vi "Initialize.vi"(0 "VISA Resource Name":refnum<visa-resource-name>, 5 "ID Query? (T: Yes)":bool=TRUE, 7 "Reset? (T: Yes)":bool=TRUE, 9 "Serial Configuration":T1={"Baud Rate (9600)"=9600, "Flow Control (2: RTS/CTS)"=2, "Parity (0: None)"=0, "Data Bits (7)"=7, "Stop Bits (10: 1.0)"=10} {"Stop Bits (10: 1.0)" items=["1.0"=10, "1.5"=15, "2.0"=20]; "Data Bits (7)" items=["7"=7, "8"=8]; "Parity (0: None)" items=["None", "Odd", "Even", "Mark", "Space"]; "Flow Control (2: RTS/CTS)" items=["None"=0, "XON/XOFF"=1, "RTS/CTS"=2, "DTR/DSR"=4]; "Baud Rate (9600)" items=["300"=300, "600"=600, "1200"=1200, "2400"=2400, "4800"=4800, "9600"=9600, "19200"=19200]}, 11 "error in (no error)":errorcluster {"code" format="%.0x"}) -> (4 "VISA Resource Name Out":refnum<visa-resource-name>, 15 "error out":errorcluster {"code" format="%.0x"})   [LabVIEW 2014, in "Agilent ESG Series.lvlib"]
doc: "This VI passes the addressing information in the instrument decriptor to the Instr Open VI and returns the instrument ID. You can optionally reset the instrument by setting the front panel reset control. You must run this VI before using any of the instrument driver VIs for this instrument."
uses:
  Agilent ESG Series.lvlib
panel:
  # "(c) 2005 - 2013 National Instruments.  ALL RIGHTS RESERVED."
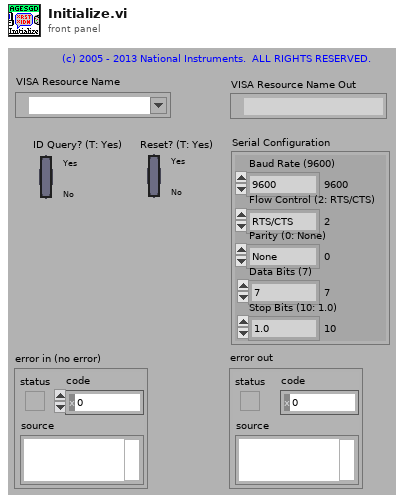
[diagram p1: front panel]
types:
  T1 = cluster{"Baud Rate (9600)":u32, "Flow Control (2: RTS/CTS)":u16, "Parity (0: None)":u16, "Data Bits (7)":u16, "Stop Bits (10: 1.0)":u16}
  T2 = cluster{"status":bool, "code":i32, "VI Name":string}
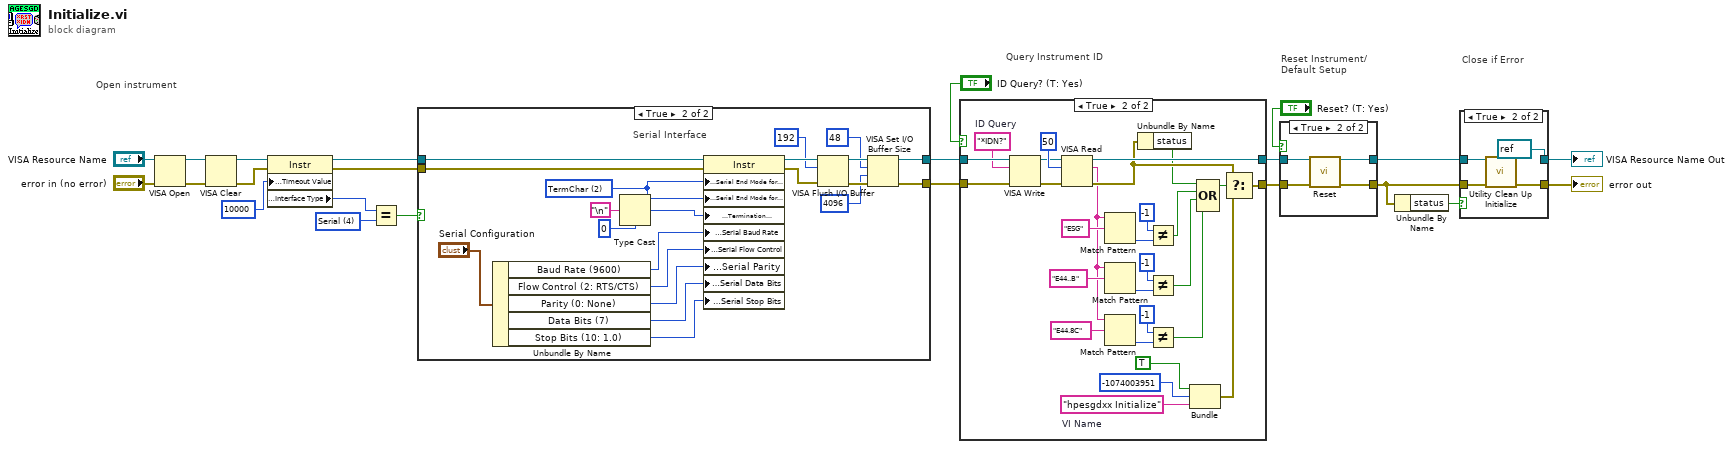
[diagram p0: block diagram]
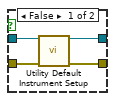
[diagram p4: hidden frame]
diagram:
  w3 = u16 4 items=["GPIB"=1, "VXI"=2, "GPIB-VXI"=3, "Serial"=4, "PXI"=5, "TCPIP"=6, "USB"=7] ("Interface Information:Interface Type")
  # "Close if Error"
  # "Query Instrument ID"
  # "Reset Instrument/\nDefault Setup"
  # "Open instrument"
  n1 = VISA Open(error in (no error)="error in (no error)", VISA resource name="VISA Resource Name") -> (VISA resource name=w10:refnum<visa-resource-name>, error out=w9:errorcluster)  [unwired: 3 in]
  n2 = VISA Clear(VISA resource name=w10, error in (no error)=w9) -> (VISA resource name out=w12:refnum<visa-resource-name>, error out=w11:errorcluster)
  n3 = property class="Instr"(reference=w12, error in=w11, "General Settings:Timeout Value"=u32 10000 ("Tmo Value")) -> (reference out=w7:refnum<visa-resource-name>, error out=w4:errorcluster, "Interface Information:Interface Type"=w2:u16)
  n4 = Equal?(x=w2, y=w3) -> (x = y?=w1:bool)
  n5 = case shown="True" w1 {
    tunnel: [w24 w43] -> w6
    tunnel: [w25 w40] -> w5
    tunnel: w7 -> [w24 w45]
    tunnel: w4 -> [w25 w46]
    frame False {
      # "GPIB, TCP/IP, and USB Interface"
    }
    frame True {
      w33 = u16 2 items=["None", "LastBit", "TermChar"] ("Serial Settings:Serial End Mode for Reads")
      # "Serial Interface"
      n6 = Unbundle By Name("Serial Configuration") -> ("Baud Rate (9600)"=w30:u32, "Flow Control (2: RTS/CTS)"=w29:u16, "Parity (0: None)"=w26:u16, "Data Bits (7)"=w28:u16, "Stop Bits (10: 1.0)"=w27:u16)
      n7 = Type Cast(type=u8 0, x="\n" ("Line Feed Constant")) -> (*(type *) &x=w32:u8)
      n8 = property class="Instr"(reference=w45, error in=w46, "Serial Settings:Serial End Mode for Reads"=w33, "Serial Settings:Serial End Mode for Writes"=w33, "Message Based Settings:Termination Character"=w32, "Serial Settings:Serial Baud Rate"=w30, "Serial Settings:Serial Flow Control"=w29, "Serial Settings:Serial Parity"=w26, "Serial Settings:Serial Data Bits"=w28, "Serial Settings:Serial Stop Bits"=w27) -> (reference out=w39:refnum<visa-resource-name>, error out=w42:errorcluster)
      n9 = VISA Flush I/O Buffer(VISA resource name=w39, mask (16)=u16 192, error in (no error)=w42) -> (VISA resource name out=w44:refnum<visa-resource-name>, error out=w41:errorcluster)
      n10 = VISA Set I/O Buffer Size(VISA resource name=w44, mask (16)=u16 48, size (4096)=u32 4096 ("size (0)"), error in (no error)=w41) -> (VISA resource name out=w43:refnum<visa-resource-name>, error out=w40:errorcluster)
    }
  }
  n11 = case shown="True" "ID Query? (T: Yes)" {
    tunnel: [w47 w76] -> w22
    tunnel: [w48 w73] -> w23
    tunnel: w6 -> [w48 w74]
    tunnel: w5 -> [w47 w75]
    frame False {
    }
    frame True {
      w69 = "*IDN?"  # ID Query
      w61 = "hpesgdxx Initialize"  # VI Name
      n12 = VISA Write(VISA resource name=w74, write buffer=w69, error in (no error)=w75) -> (VISA resource name out=w62:refnum<visa-resource-name>, error out=w64:errorcluster)  [unwired: 1 out]
      n13 = VISA Read(VISA resource name=w62, byte count=u32 50, error in (no error)=w64) -> (VISA resource name out=w73:refnum<visa-resource-name>, read buffer=w49:string, error out=w63:errorcluster)  [unwired: 1 out]
      n14 = Match Pattern(string=w49, regular expression="ESG") -> (offset past match=w67:i32)  [unwired: 1 in, 3 out]
      n15 = Match Pattern(string=w49, regular expression="E44..B") -> (offset past match=w55:i32)  [unwired: 1 in, 3 out]
      n16 = Match Pattern(string=w49, regular expression="E44.8C") -> (offset past match=w53:i32)  [unwired: 1 in, 3 out]
      n17 = Unbundle By Name(w63) -> ("status"=w60:bool)
      n18 = Not Equal?(x=-1, y=w67) -> (x != y?=w59:bool)
      n19 = Not Equal?(x=-1, y=w55) -> (x != y?=w54:bool)
      n20 = Not Equal?(x=-1, y=w53) -> (x != y?=w50:bool)
      n21 = Bundle(TRUE, -1074003951, "VI Name"=w61) -> (w70:cluster{bool, i32, "VI Name":string})  [unwired: 1 in]
      n22 = Compound Arithmetic op=OR(w60, w59, w54, w50) -> (w58:bool)
      n23 = Select(t=w63, s=w58, f=w70) -> (s? t:f=w76:T2)
    }
  }
  n24 = case shown="True" "Reset? (T: Yes)" {
    tunnel: w22 -> [w79 w81]
    tunnel: [w78 w84] -> w19
    tunnel: w23 -> [w80 w82]
    tunnel: [w77 w83] -> w18
    frame False {
      n25 = call "Utility Default Instrument Setup.vi"("VISA Resource Name"=w80, "error in (no error)"=w79) -> ("VISA Resource Name Out"=w77:refnum<visa-resource-name>, "error out"=w78:errorcluster)  [unwired: 12 in]
    }
    frame True {
      n26 = call "Reset.vi"("VISA Resource Name"=w82, "error in (no error)"=w81) -> ("VISA Resource Name Out"=w83:refnum<visa-resource-name>, "error out"=w84:errorcluster)  [unwired: 12 in]
    }
  }
  n27 = Unbundle By Name(w19) -> ("status"=w20:bool)
  n28 = case shown="True" w20 {
    tunnel: w18 -> [w86 w90]
    tunnel: w19 -> [w85 w89]
    tunnel: [w86 refnum<visa-resource-name> refnum ("VISA Resource Name Out")] -> w14
    tunnel: [w85 w88] -> w17
    frame False {
    }
    frame True {
      n29 = call "Utility Clean Up Initialize.vi"("VISA session"=w90, "error in (no error)"=w89) -> ("error out"=w88:errorcluster)  [unwired: 13 in]
    }
  }
  "error out" <- w17
  "VISA Resource Name Out" <- w14
